vi "MIF_N_txt-de-obs.vi"(9 "xt obs":string[](array[string]), 11 "xt mif":string[](array[string])) -> (2 "ni-mif":i32[](array[numeric]))   [LabVIEW 2010, in "lv_02.lvlib"]
uses:
  lv_02.lvlib
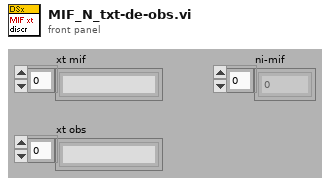
[diagram p1: front panel]
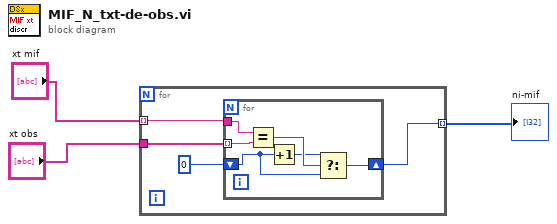
[diagram p0: block diagram]
diagram:
  n1 = for {
    tunnel: "xt mif" -> [w7] mode=indexing
    tunnel: "xt obs" -> [w6]
    tunnel: [w4] -> w3 mode=indexing
    n2 = for {
      tunnel: w7 -> [w13]
      tunnel: w6 -> [w8] mode=indexing
      shift-right: [w12] -> w4
      shift-left: 0 -> [w9]
      n3 = Equal?(x=w13, y=w8) -> (x = y?=w11:bool)
      n4 = Increment(x=w9) -> (x+1=w10:i32)
      n5 = Select(t=w10, s=w11, f=w9) -> (s? t:f=w12:i32)
    }
  }
  "ni-mif" <- w3
